vi "CANOpen Edit SDOs - List.vi"(8 "error in (no error)":errorcluster, 11 "Node Ptr":u64 format="%.0x") -> ()   [LabVIEW 2021, in "CANOpen Addon System Explorer.lvlib"]
uses:
  CANOpen Addon System Explorer.lvlib
  Shared/CANOpen_SDO Settings.ctl
  Shared/CANOpen Addon GUID Lookup Global.vi
  <vilib>/NI VeriStand/Custom Device API/Get Item Property (Variant).vi
  <vilib>/NI VeriStand/Custom Device API/Set Item Property (Variant).vi
  <vilib>/NI VeriStand/Custom Device API/Custom Device API.lvlib
  Shared/CANOpen Addon Shared.lvlib
  <vilib>/NI VeriStand/Custom Device Tools/Custom Device Utility Library/Custom Device Utility Library.lvlib
panel:
  out "error out":errorcluster
  in  "Tag":string
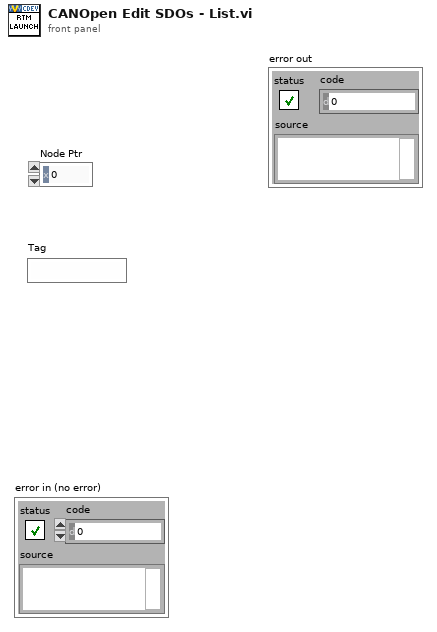
[diagram p1: front panel]
types:
  T1 = typedef "CANOpen Addon Shared.lvlib/CANOpen_SDO Settings.ctl" = cluster{"Object Index":u16, "Sub-Index (0)":u8, "Block Data":u8[], "Name":string}
  T2 = typedef "Custom Device API.lvlib/Custom Device Item Ref.ctl" = u64
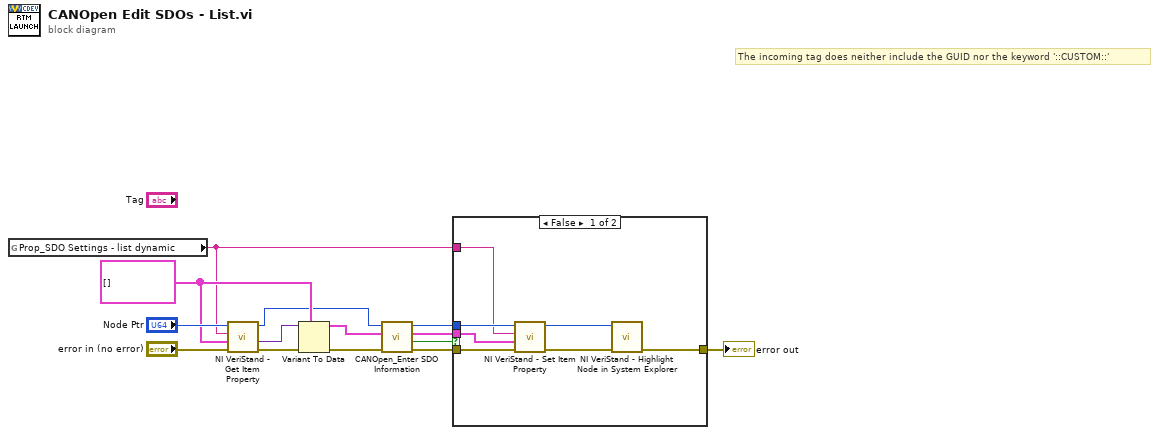
[diagram p0: block diagram]
diagram:
  w10 = T1[] [] ("SDO Parameters")
  # "The incoming tag does neither include the GUID nor the keyword '::CUSTOM::'"
  n1 = global read "CANOpen Addon GUID Lookup Global.vi" "Prop_SDO Settings - list dynamic"() -> (w2:string)
  n2 = call-poly <vilib>:"NI VeriStand - Get Item Property.vi"("error in (no error)"="error in (no error)", "Default Value"=w10, "Property Name"=w2, "Item Ref in"="Node Ptr") -> ("error out"=w14:errorcluster, "Value"=w13:variant, "Item Ref out"=w7:T2)  [unwired: 4 in, 1 out]
  n3 = Variant To Data(error in=w14, type=w10, Variant=w13) -> (data=w9:T1[], error out=w8:errorcluster)
  n4 = call "CANOpen_Enter SDO Information.vi"("error in (no error)"=w8, "SDO Parameters"=w9, "Node Ptr"=w7) -> ("error out"=w5:errorcluster, "Cancelled?"=w6:bool, "SDO Parameters"=w4:T1[], "Item Ref out"=w3:T2)  [unwired: 5 in]
  n5 = case shown="False" w6 {
    tunnel: w5 -> [w21 w22]
    tunnel: w3 -> [w19 _]
    tunnel: w4 -> [w20 _]
    tunnel: [w16 w22] -> w1
    tunnel: w2 -> [w18 _]
    frame False {
      n6 = call-poly <vilib>:"NI VeriStand - Set Item Property.vi"("error in (no error)"=w21, "Value"=w20, "Property Name"=w18, "Item Ref in"=w19) -> ("error out"=w17:errorcluster, "Item Ref out"=w15:T2)  [unwired: 5 in, 1 out]
      n7 = call <vilib>:"NI VeriStand - Highlight Node in System Explorer.vi"("error in (no error)"=w17, "Item Ref in"=w15) -> ("error out"=w16:errorcluster)  [unwired: 8 in, 1 out]
    }
    frame True {
    }
  }
  "error out" <- w1
